vi "Remove Duplicates.vi"(8 "error in (no error)":errorcluster, 11 "Dynamic Member VIs":refnum<vi>[](array[refnum])) -> (0 "error out":errorcluster, 3 "Unique Dynamic Member VIs":refnum<vi>[](array[refnum]))   [LabVIEW 2020, in "Mock Class Generator.lvclass"]
uses:
  Mock Class Generator.lvclass
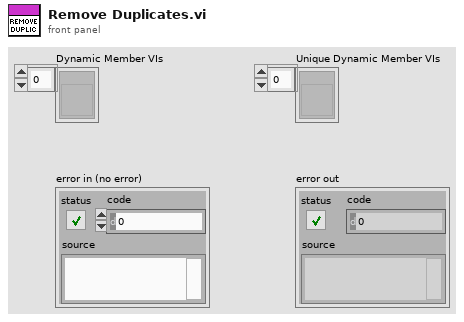
[diagram p1: front panel]
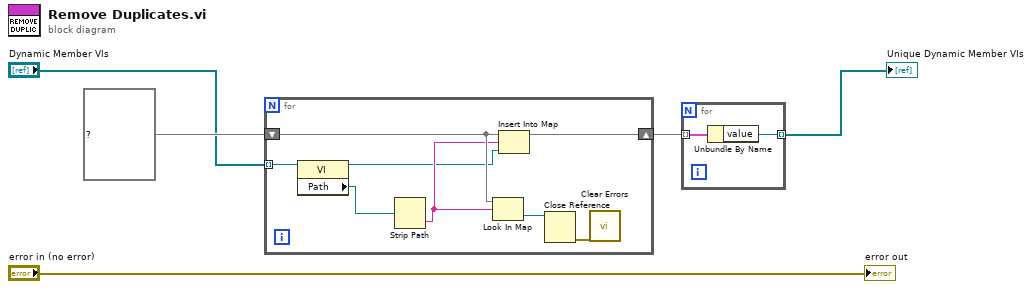
[diagram p0: block diagram]
diagram:
  n1 = for {
    tunnel: "Dynamic Member VIs" -> [w13] mode=indexing
    shift-right: [w11] -> w3
    shift-left: map{string, refnum<vi>} {} ("map") -> [w10]
    n2 = property class="VI"(reference=w13) -> (reference out=w6:refnum<vi>, "Path"=w12:path)  [unwired: 1 in, 1 out]
    n3 = Strip Path(path=w12) -> (name=w7:string)  [unwired: 1 out]
    n4 = Look In Map(map=w10, key=w7) -> (value=w9:refnum<vi>)  [unwired: 1 in, 1 out]
    n5 = Insert Into Map(map in=w10, key=w7, value=w6) -> (map out=w11:map{string, refnum<vi>})  [unwired: 2 out]
    n6 = Close Reference(reference=w9) -> (error out=w8:errorcluster)  [unwired: 1 in]
    n7 = call <vilib>:"Clear Errors.vi"("error in (no error)"=w8) -> ()  [unwired: 5 in, 2 out]
  }
  n8 = for {
    tunnel: w3 -> [w15] mode=indexing
    tunnel: [w14] -> w1 mode=indexing
    n9 = Unbundle By Name(w15) -> ("value"=w14:refnum<vi>)
  }
  "Unique Dynamic Member VIs" <- w1
  "error out" <- "error in (no error)"
